vi "After Launch Init Core.vi"(8 "error in (no error)":errorcluster, 11 "CS++ControllerActor in":refnum<class "CS++ControllerActor.lvclass">) -> (0 "error out":errorcluster, 3 "CS++ControllerActor out":refnum<class "CS++ControllerActor.lvclass">)   [LabVIEW 2014, in "CS++ControllerActor.lvlib" / "CS++ControllerActor.lvclass"]
doc: "Use <b>Pre Launch init.vi</b> method only for sanity checks that are supposed to prevent the actor from launching if they fail. Use <B>this</B> method instead to initialize unique resources that must be released during the <b>Stop Core.vi</b> method. A corresponding high priority message will become dispatched before the <B>Actor Framework.lvlib:Actor.lvclass.Actor Core.vi</b> is called.\n\n<b>Derived classed should call the parent methode first</b> and their own initialization code after.\n\nRefer also to the ongoing discussion at https://decibel.ni.com/content/message/57394#57394."
uses:
  CS++ControllerActor.lvclass
  CS++ControllerActor Messages/Register PVs Msg/Register PVs Msg.lvclass
  CS++BaseActor/CS++BaseActor.lvclass/CS++BaseActor.ctl
  CS++ControllerActor.lvclass/CS++ControllerActor.ctl
  CS++PVMonitor Messages/CS++PVUpdate Msg/CS++PVUpdate Msg.lvclass
  CS++PVMonitor Messages/CS++PVUpdate Msg/CS++PVUpdate Msg.lvclass/CS++PVUpdate Msg.ctl
  Classes/CS++ProcessVariables/ProcessVariable/PV.lvclass/PV.ctl
  Classes/CS++ProcessVariables/ProcessVariable/PV.lvclass
  <vilib>/ActorFramework/Actor/Actor.lvclass/Actor.ctl
  <vilib>/ActorFramework/Message Enqueuer/Message Enqueuer.lvclass/Message Enqueuer.ctl
  CS++BaseActor Messages/Launch Associated GUI Msg/Launch Associated GUI Msg.lvclass/Launch Associated GUI Msg.ctl
  Classes/CS++ProcessVariables/ProcessVariable/Write Data.vi
  Classes/CS++ProcessVariables/ProcessVariable/Write Timestamp.vi
  Classes/CS++ProcessVariables/ProcessVariable/Write Quality.vi
  Classes/CS++ProcessVariables/ProcessVariable/Write status.vi
  Classes/CS++ProcessVariables/ProcessVariable/Write Type Descriptor.vi
  Classes/CS++ProcessVariables/ProcessVariable/Write PV URL.vi
  Classes/CS++ProcessVariables/ProcessVariable/Write Name.vi
  Classes/CS++ProcessVariables/ProcessVariable/Read PV URL.vi
  <vilib>/ActorFramework/Message Enqueuer/Init from Existing Queue.vi
  <vilib>/ActorFramework/Message Enqueuer/Enqueue.vi
  <vilib>/ActorFramework/Message Priority Queue/Priority Enqueue.vi
  CS++BaseActor/CS++BaseActor.lvclass
  CS++BaseActor Messages/Launch Associated GUI Msg/Launch Associated GUI Msg.lvclass
  <vilib>/ActorFramework/Message Enqueuer/Message Enqueuer.lvclass
  Classes/CS++BaseClasses/Factory/CS++Factory.lvclass
  <vilib>/ActorFramework/Actor/Actor.lvclass
  Classes/CS++ProcessVariables/PVConnection/PVConnection.lvclass
  Classes/CS++ProcessVariables/CS++ProcessVariables.lvlib
  Libraries/Utilities/CS++Utilities.lvlib
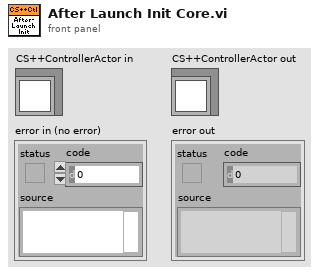
[diagram p1: front panel]
types:
  T1 = cluster{"Name":string, "Polling-String":string, "CS++PVUpdate Msg":refnum<class "CS++PVUpdate Msg.lvclass">, "PVConnection":refnum<class "PVConnection.lvclass">}[]
  T2 = cluster{"Name":string, "Polling-String":string, "CS++PVUpdate Msg out":refnum<class "CS++PVUpdate Msg.lvclass">, "PVConnection":refnum<class "PVConnection.lvclass">}
  T3 = cluster{"Name":string, "Polling-String":string, "CS++PVUpdate Msg out":refnum<class "CS++PVUpdate Msg.lvclass">, "PVConnection":refnum<class "PVConnection.lvclass">}[]
  T4 = cluster{"Read Access":enum8{"Allowed", "Required", "None"}, "Write Access":enum8{"Allowed", "Required", "None"}}
  T5 = cluster{"Name":string, "Polling-String":string, "CS++PVUpdate Msg":refnum<class "CS++PVUpdate Msg.lvclass">, "PVConnection":refnum<class "PVConnection.lvclass">}
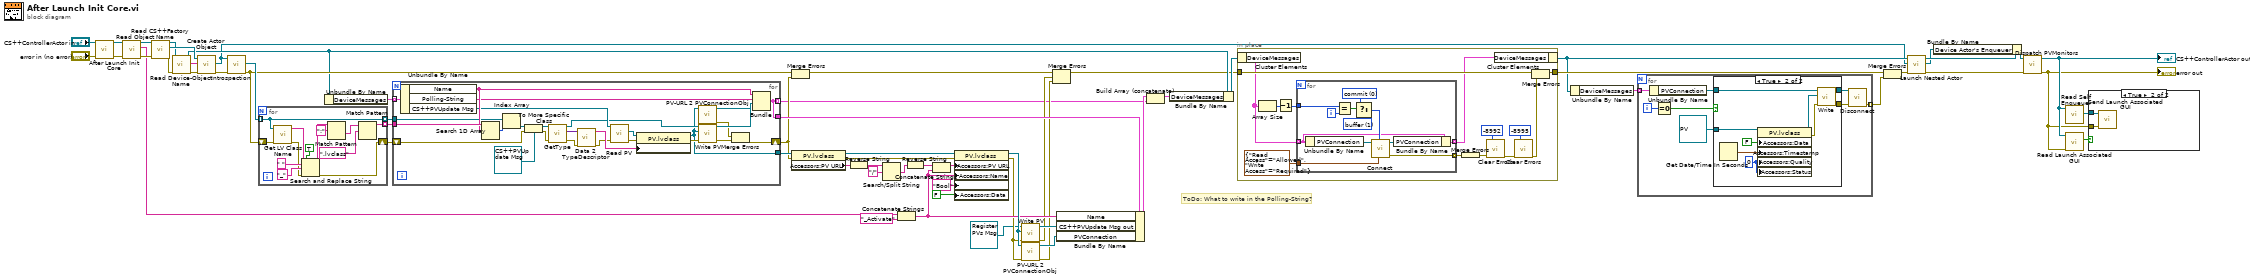
[diagram p0: block diagram]
diagram:
  # "ToDo: What to write in the Polling-String?"
  n1 = call-parent "After Launch Init Core.vi"("error in (no error)"="error in (no error)", "CS++BaseActor in"="CS++ControllerActor in") -> ("error out"=w26:errorcluster, "CS++BaseActor out"=w27:refnum<class "CS++ControllerActor.lvclass">)  [unwired: 8 in]
  n2 = call "Read Object Name.vi"("error in (no error)"=w26, "CS++BaseActor in"=w27) -> ("error out"=w29:errorcluster, "Object Name"=w25:string, "CS++BaseActor out"=w28:refnum<class "CS++ControllerActor.lvclass">)  [unwired: 7 in]
  n3 = call "Read CS++Factory.vi"("error in (no error)"=w29, "CS++BaseActor in"=w28) -> ("error out"=w59:errorcluster, "CS++Factory"=w60:refnum<class "CS++Factory.lvclass">, "CS++BaseActor out"=w57:refnum<class "CS++ControllerActor.lvclass">)  [unwired: 7 in]
  n4 = call-dynamic "Read Device-Object Name.vi"("error in (no error)"=w59, "CS++ControllerActor in"=w57) -> ("error out"=w58:errorcluster, "Device-Object Name"=w56:string, "CS++ControllerActor out"=w45:refnum<class "CS++ControllerActor.lvclass">)  [unwired: 7 in]
  n5 = call "Create Actor Object.vi"("error in (no error)"=w58, "Object Name"=w56, "CS++Factory in"=w60) -> ("error out"=w44:errorcluster, "CS++BaseActor"=w40:refnum<class "CS++BaseActor.lvclass">)  [unwired: 5 in, 2 out]
  n6 = call "Introspection.vi"("error in (no error)"=w44, "CS++BaseActor in"=w40) -> ("error out"=w46:errorcluster, "CS++Messages"=w51:refnum<class "Message.lvclass">[])  [unwired: 7 in, 1 out]
  n7 = for {
    tunnel: w51 -> [w75] mode=indexing
    tunnel: [w75] -> w50 mode=indexing
    tunnel: [w64] -> w49 mode=indexing
    shift-right: [w68] -> w48
    shift-left: w46 -> [w74]
    n8 = call <vilib>:"Get LV Class Name.vi"("error in (no error)"=w74, "object"=w75) -> ("error out"=w69:errorcluster, "class name"=w73:string)  [unwired: 8 in]
    n9 = Search and Replace String(replace all?=TRUE ("Replace All? (false)"), input string=w73, search string=" ", replace string="_" ("Replace Pattern (\"\")"), error in=w69) -> (result string=w67:string, error out=w68:errorcluster)  [unwired: 3 in, 2 out]
    n10 = Match Pattern(string=w67, regular expression=":") -> (after substring=w65:string)  [unwired: 1 in, 3 out]
    n11 = Match Pattern(string=w65, regular expression=".lvclass") -> (before substring=w64:string)  [unwired: 1 in, 3 out]
  }
  n12 = Unbundle By Name(w45) -> ("DeviceMessages"=w52:T1)
  n13 = for {
    tunnel: w52 -> [w102] mode=indexing
    tunnel: w50 -> [w99]
    tunnel: w49 -> [w101]
    tunnel: [w77] -> w2 mode=indexing
    shift-right: [w87] -> w21
    shift-left: w48 -> [w95]
    tunnel: [w77] -> w32
    tunnel: [w76] -> w22
    n14 = Unbundle By Name(w102) -> ("Name"=w100:string, "Polling-String"=w97:string, "CS++PVUpdate Msg"=w80:refnum<class "CS++PVUpdate Msg.lvclass">)
    n15 = Search 1D Array(1D array=w101, element=w100) -> (index of element=w98:i32)  [unwired: 1 in]
    n16 = Index Array(array=w99, index=w98) -> (element=w96:refnum<class "Message.lvclass">)
    n17 = To More Specific Class(target class=refnum<class "CS++PVUpdate Msg.lvclass"> refnum ("CS++PVMonitor.lvlib:CS++PVUpdate Msg.lvclass"), reference=w96, error in=w95) -> (specific class reference=w86:refnum<class "CS++PVUpdate Msg.lvclass">, error out=w85:errorcluster)
    n18 = call-dynamic "GetType.vi"("error in (no error)"=w85, "CS++PVUpdate Msg in"=w86) -> ("error out"=w81:errorcluster, "Data Sample"=w84:variant, "CS++PVUpdate Msg out"=w79:refnum<class "CS++PVUpdate Msg.lvclass">)  [unwired: 7 in]
    n19 = call "Data 2 TypeDescriptor.vi"("error in (no error)"=w81, "Data"=w84) -> ("Error Out"=w82:errorcluster, "TypeDescriptor"=w83:string)  [unwired: 8 in]
    n20 = call "Read PV.vi"("error in (no error)"=w82, "CS++PVUpdate Msg in"=w80) -> ("error out"=w92:errorcluster, "PV"=w93:refnum<class "PV.lvclass">)  [unwired: 7 in, 1 out]
    n21 = property class="PV.lvclass"(reference=w93, error in=w92, "Accessors:Type Descriptor"=w83) -> (reference out=w76:refnum<class "PV.lvclass">, error out=w91:errorcluster)
    n22 = call "PV-URL 2 PVConnectionObj.vi"("PV"=w76) -> ("Error Out"=w88:errorcluster, "PVConnection"=w90:refnum<class "PVConnection.lvclass">)  [unwired: 8 in, 1 out]
    n23 = call "Write PV.vi"("error in (no error)"=w91, "PV"=w76, "CS++PVUpdate Msg in"=w79) -> ("error out"=w89:errorcluster, "CS++PVUpdate Msg out"=w94:refnum<class "CS++PVUpdate Msg.lvclass">)  [unwired: 7 in]
    n24 = Merge Errors(w88, w89) -> (w87:errorcluster)
    n25 = Bundle("Name"=w100, "Polling-String"=w97, "CS++PVUpdate Msg out"=w94, "PVConnection"=w90) -> (w77:T2)  [unwired: 1 in]
  }
  n26 = Merge Errors(w46, w21) -> (w8:errorcluster)
  n27 = property class="PV.lvclass"(reference=w22, error in=w21) -> (reference out=w13:refnum<class "PV.lvclass">, error out=w12:errorcluster, "Accessors:PV URL"=w18:string)
  n28 = Reverse String(1:w18) -> (0:w17:string)
  n29 = Search/Split String(string=w17, search string/char (-)="/") -> (match + rest of string=w15:string)  [unwired: 1 in, 2 out]
  n30 = Concatenate Strings(w25, "_Activate" ("string")) -> (w10:string)
  n31 = Reverse String(1:w15) -> (0:w14:string)
  n32 = Concatenate Strings(w14, w10) -> (w11:string)
  n33 = property class="PV.lvclass"(reference=w13, error in=w12, "Accessors:PV URL"=w11, "Accessors:Name"=w10, "Accessors:Type Descriptor"="Bool" ("Type Descriptor"), "Accessors:Data"=FALSE) -> (reference out=w23:refnum<class "PV.lvclass">, error out=w9:errorcluster)
  n34 = call "Write PV.vi"("error in (no error)"=w9, "PV"=w23, "CS++PVUpdate Msg in"=refnum<class "Register PVs Msg.lvclass"> refnum ("CS++ControllerActor.lvlib:Register PVs Msg.lvclass")) -> ("error out"=w6:errorcluster, "CS++PVUpdate Msg out"=w31:refnum<class "Register PVs Msg.lvclass">)  [unwired: 7 in]
  n35 = call "PV-URL 2 PVConnectionObj.vi"("Error In"=w9, "PV"=w23) -> ("Error Out"=w5:errorcluster, "PVConnection"=w30:refnum<class "PVConnection.lvclass">)  [unwired: 7 in, 1 out]
  n36 = Merge Errors(w8, w6, w5) -> (w7:errorcluster)
  n37 = Bundle By Name(cluster=w32, "Name"=w10, "CS++PVUpdate Msg out"=w31, "PVConnection"=w30) -> (w3:T2)
  n38 = Build Array (concatenate)(w3, w2) -> (w19:T3)
  n39 = Bundle By Name(cluster=w45, "DeviceMessages"=w19) -> (w47:refnum<class "CS++ControllerActor.lvclass">)
  n40 = in-place {
    in-place-border: [w115] -> w54
    in-place-border: w7 -> [w114]
    n41 = in-place-cluster #1(w47) -> ("DeviceMessages"=w111:T1)
    n42 = Array Size(array=w111) -> (size(s)=w110:i32)
    n43 = Decrement(x=w110) -> (x-1=w109:i32)
    n44 = for {
      tunnel: w111 -> [w118] mode=indexing
      tunnel: [w117] -> w113 mode=indexing
      tunnel: T4 {"Read Access"=enum."Allowed", "Write Access"=enum."Required"} ("Access (R/W allowed)") -> [w127]
      tunnel: [w126] -> w106 mode=indexing
      tunnel: w109 -> [w124]
      i -> [w125]
      w121 = u16 1 items=["commit", "buffer"] ("Mode (commit)")
      w122 = u16 0 items=["commit", "buffer"] ("Mode (commit)")
      n45 = Unbundle By Name(w118) -> ("PVConnection"=w119:refnum<class "PVConnection.lvclass">)
      n46 = Equal?(x=w124, y=w125) -> (x = y?=w123:bool)
      n47 = Select(t=w122, s=w123, f=w121) -> (s? t:f=w120:u16)
      n48 = call "Connect.vi"("Access (R/W allowed)"=w127, "Mode (buffer)"=w120, "PVConnection in"=w119) -> ("Error Out"=w126:errorcluster, "PVConnection out"=w116:refnum<class "PVConnection.lvclass">)  [unwired: 7 in]
      n49 = Bundle By Name(cluster=w118, "PVConnection"=w116) -> (w117:T5)
    }
    n50 = Merge Errors(w106) -> (w104:errorcluster)
    n51 = call <vilib>:"Clear Errors.vi"("error in (no error)"=w104, "specific error code to clear (0: all)"=-8992) -> ("error out"=w103:errorcluster)  [unwired: 4 in, 1 out]
    n52 = in-place-cluster #1("DeviceMessages"=w113) -> (w42:refnum<class "CS++ControllerActor.lvclass">)
    n53 = call <vilib>:"Clear Errors.vi"("error in (no error)"=w103, "specific error code to clear (0: all)"=-8995) -> ("error out"=w108:errorcluster)  [unwired: 4 in, 1 out]
    n54 = Merge Errors(w114, w108) -> (w115:errorcluster)
  }
  n55 = Unbundle By Name(w42) -> ("DeviceMessages"=w55:T1)
  n56 = for {
    tunnel: w55 -> [w134] mode=indexing
    tunnel: [w135] -> w53 mode=indexing
    i -> [w131]
    n57 = Unbundle By Name(w134) -> ("PVConnection"=w133:refnum<class "PVConnection.lvclass">)
    n58 = Equal To 0?(x=w131) -> (x = 0?=w130:bool)
    n59 = case shown="True" w130 {
      tunnel: w133 -> [w136 w145]
      tunnel: [w136 w144] -> w132
      tunnel: refnum<class "PV.lvclass"> refnum ("CS++ProcessVariables.lvlib:PV.lvclass") -> [_ w143]
      tunnel: [_ w140] -> w128
      frame False {
      }
      frame True {
        w137 = 0 ("Quality")
        n60 = Get Date/Time In Seconds() -> (seconds since 1Jan1904=w139:timestamp)
        n61 = property class="PV.lvclass"(reference=w143, "Accessors:Data"=FALSE, "Accessors:Timestamp"=w139, "Accessors:Quality"=w137, "Accessors:Status"=w137) -> (reference out=w142:refnum<class "PV.lvclass">, error out=w141:errorcluster)  [unwired: 1 in]
        n62 = call "Write.vi"("error in (no error)"=w141, "PV"=w142, "PVConnection in"=w145) -> ("error out"=w140:errorcluster, "PVConnection out"=w144:refnum<class "PVConnection.lvclass">)  [unwired: 7 in]
      }
    }
    n63 = call "Disconnect.vi"("error in (no error)"=w128, "PVConnection in"=w132) -> ("error out"=w135:errorcluster)  [unwired: 8 in, 1 out]
  }
  n64 = Merge Errors(w54, w53) -> (w43:errorcluster)
  n65 = call <vilib>:"Launch Nested Actor.vi"("error in (no error)"=w43, "Nested Actor"=w40, "Caller Actor in"=w42) -> ("error out"=w41:errorcluster, "Nested Actor's Enqueuer"=w37:refnum<class "Message Enqueuer.lvclass">, "Caller Actor out"=w39:refnum<class "CS++ControllerActor.lvclass">)  [unwired: 6 in]
  n66 = Bundle By Name(cluster=w39, "Device Actor's Enqueuer"=w37) -> (w38:refnum<class "CS++ControllerActor.lvclass">)
  n67 = call "Dispatch PVMonitors.vi"("Error In"=w41, "CS++ControllerActor in"=w38) -> ("Error Out"=w33:errorcluster, "CS++ControllerActor out"=w34:refnum<class "CS++ControllerActor.lvclass">)  [unwired: 8 in]
  "error out" <- w33
  "CS++ControllerActor out" <- w34
  n68 = call <vilib>:"Read Self Enqueuer.vi"("Actor"=w34) -> ("Self Enqueuer"=w36:refnum<class "Message Enqueuer.lvclass">)  [unwired: 10 in]
  n69 = call "Read Launch Associated GUI.vi"("error in (no error)"=w33, "CS++BaseActor in"=w34) -> ("Launch Associated GUI"=w35:bool)  [unwired: 7 in, 2 out]
  n70 = case shown="True" w35 {
    tunnel: w36 -> [_ w147]
    tunnel: w33 -> [_ w146]
    frame False {
    }
    frame True {
      n71 = call "Send Launch Associated GUI.vi"("error in (no error)"=w146, "Message Enqueuer"=w147) -> ()  [unwired: 8 in, 2 out]
    }
  }
